vi "Update User Interface.vi"(8 "error in (no error)":errorcluster, 9 "VI Refnum":refnum<vi>, 11 "Data In":T1 {"Language" items=["English", "Español", "Português"]}) -> (0 "error out":errorcluster, 3 "Data Out":T1 {"Language" items=["English", "Español", "Português"]})   [LabVIEW 2017]
uses:
  Controls/HID Data.ctl
  <vilib>/userdefined/High Color/IMAQdx.ctl
  <vilib>/vision/Image Controls.llb/IMAQ Image.ctl
  Controls/HID State.ctl
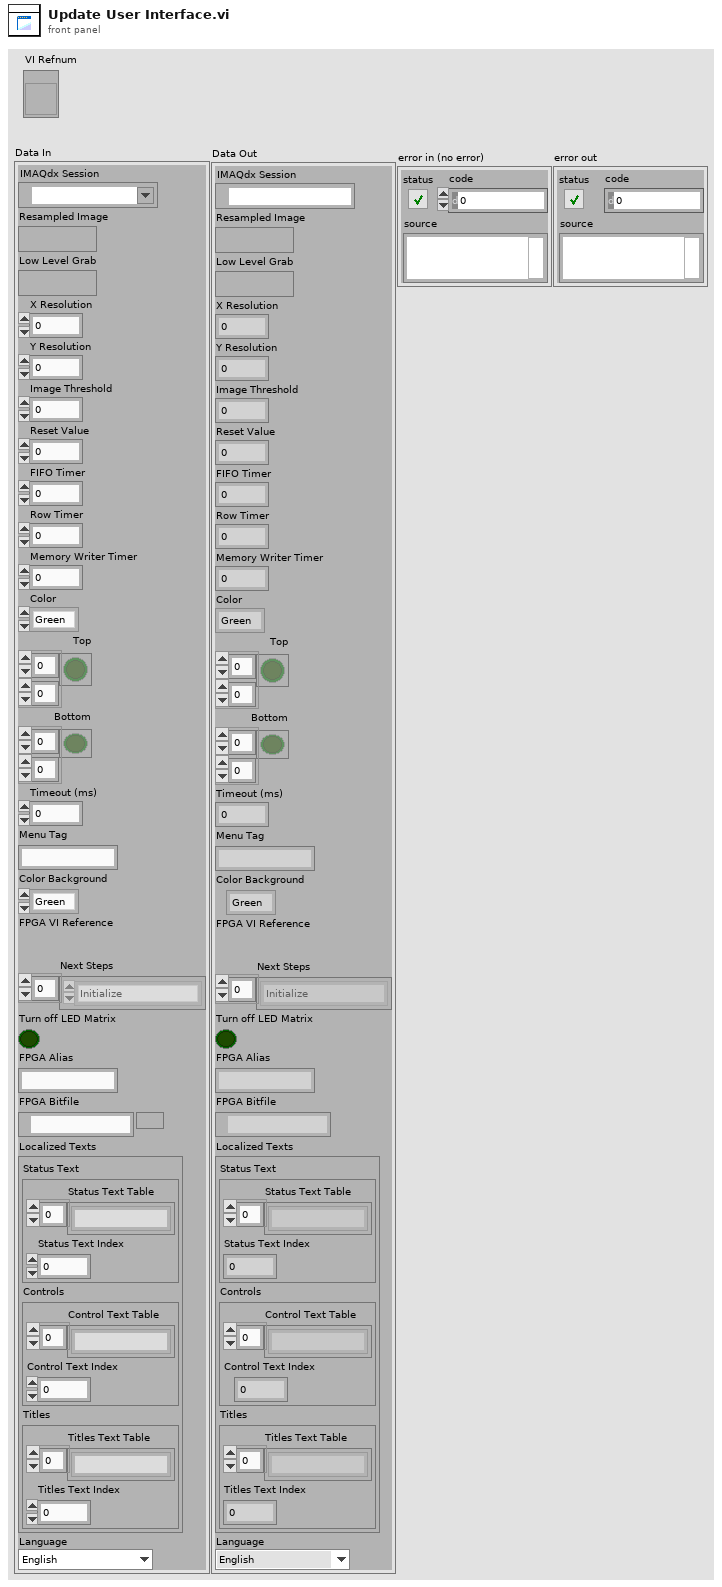
[diagram p1: front panel]
types:
  T1 = typedef "HID Data.ctl" = cluster{"IMAQdx Session":T2, "Resampled Image":T3, "Low Level Grab":T3, "X Resolution":i32, "Y Resolution":i32, "Image Threshold":u8, "Reset Value":i32, "FIFO Timer":u16, "Row Timer":u32, "Memory Writer Timer":u8, "Color":enum16{"Green", "Blue", "Red", "White", "Pink", "Yellow", "Turquoise", "Black"}, "Top":bool[][], "Bottom":bool[][], "Timeout (ms)":i32, "Menu Tag":string, "Color Background":enum16{"Green", "Blue", "Red", "White", "Pink", "Yellow", "Turquoise", "Black"}, "FPGA VI Reference":refnum<k20>, "Next Steps":T4[], "Turn off LED Matrix":bool, "FPGA Alias":string, "FPGA Bitfile":path, "Localized Texts":cluster{"Status Text":cluster{"Status Text Table":string[], "Status Text Index":i32}, "Controls":cluster{"Control Text Table":string[], "Control Text Index":i32}, "Titles":cluster{"Titles Text Table":string[], "Titles Text Index":i32}}, "Language":u16}
  T2 = typedef "IMAQdx.ctl" = refnum<k21>
  T3 = typedef "IMAQ Image.ctl" = refnum<image>
  T4 = typedef "HID State.ctl" = enum16{"Initialize", "Set FPGA Parametes", "Set Camera Parameters", "Set LED Matrix Parameters", "Initialize FPGA Interface", "Initialize Camera", "Start FPGA VI", "Start Camera", "Wait for Event", "Update UI", "Acquire", "Process Image", "Get Boolean Arrays", "Send to FPGA", "Menu Pop-Up", "Menu Actions", "Handle Errors", "Close Camera", "Close FPGA", "Stop", "Exit"}
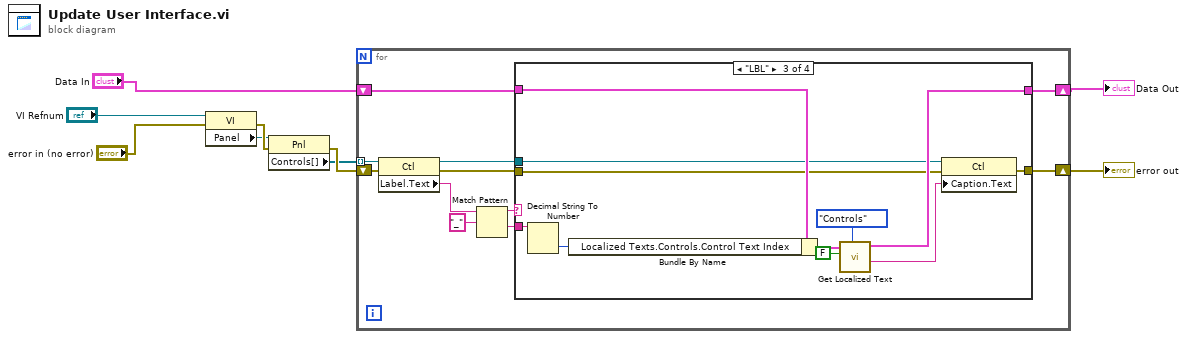
[diagram p0: block diagram]
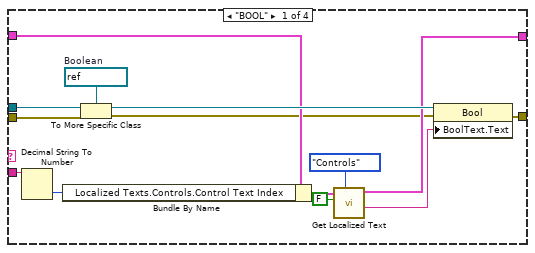
[diagram p2: hidden frame]
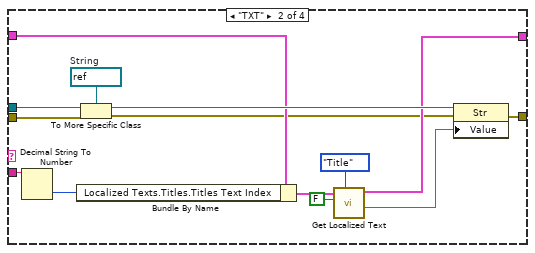
[diagram p3: hidden frame]
diagram:
  n1 = property class="VI"(reference="VI Refnum", error in="error in (no error)") -> (error out=w8:errorcluster, "Panel"=w6:refnum<vi>)  [unwired: 1 out]
  n2 = property class="Pnl"(reference=w6, error in=w8) -> (error out=w9:errorcluster, "Controls[]"=w5:refnum<vi>[])  [unwired: 1 out]
  n3 = for {
    tunnel: w5 -> [w18] mode=indexing
    shift-right: [w14] -> w3
    shift-left: "Data In" -> [w15]
    shift-right: [w11] -> w2
    shift-left: w9 -> [w10]
    n4 = property class="Ctl"(reference=w18, error in=w10) -> (reference out=w13:refnum<vi>, error out=w12:errorcluster, "Label.Text"=w17:string)
    n5 = Match Pattern(string=w17, regular expression="_") -> (before substring=w19:string, after substring=w16:string)  [unwired: 1 in, 2 out]
    n6 = case shown="\"LBL\"" w19 {
      tunnel: w16 -> [w32 w46 w59 _]
      tunnel: w15 -> [w29 w43 w56 w60]
      tunnel: [w28 w42 w55 w60] -> w14
      tunnel: w13 -> [w25 w39 w52 _]
      tunnel: w12 -> [w24 w38 w51 w61]
      tunnel: [w22 w36 w50 w61] -> w11
      frame "BOOL" {
        w33 = refnum<vi> refnum  # Boolean
        n7 = Decimal String To Number(string=w32) -> (number=w26:i32)  [unwired: 2 in, 1 out]
        n8 = Bundle By Name(cluster=w29, "Localized Texts.Controls.Control Text Index"=w26) -> (w27:T1)
        n9 = To More Specific Class(target class=w33, reference=w25, error in=w24) -> (specific class reference=w34:refnum<vi>, error out=w23:errorcluster)
        n10 = call "Get Localized Text.vi"("Text Type"=enum16{"Status", "Title", "Controls"}."Controls", "Force Index"=FALSE, "Data In"=w27) -> ("Localized Text"=w30:string, "Data Out"=w28:T1)  [unwired: 7 in]
        n11 = property class="Bool"(reference=w34, error in=w23, "BoolText.Text"=w30) -> (error out=w22:errorcluster)  [unwired: 1 out]
      }
      frame "TXT" {
        w47 = refnum<vi> refnum  # String
        n12 = Decimal String To Number(string=w46) -> (number=w40:i32)  [unwired: 2 in, 1 out]
        n13 = Bundle By Name(cluster=w43, "Localized Texts.Titles.Titles Text Index"=w40) -> (w41:T1)
        n14 = To More Specific Class(target class=w47, reference=w39, error in=w38) -> (specific class reference=w48:refnum<vi>, error out=w37:errorcluster)
        n15 = call "Get Localized Text.vi"("Text Type"=enum16{"Status", "Title", "Controls"}."Title", "Force Index"=FALSE, "Data In"=w41) -> ("Localized Text"=w44:string, "Data Out"=w42:T1)  [unwired: 7 in]
        n16 = property class="Str"(reference=w48, error in=w37, "Value"=w44) -> (error out=w36:errorcluster)  [unwired: 1 out]
      }
      frame "LBL" {
        n17 = Decimal String To Number(string=w59) -> (number=w53:i32)  [unwired: 2 in, 1 out]
        n18 = Bundle By Name(cluster=w56, "Localized Texts.Controls.Control Text Index"=w53) -> (w54:T1)
        n19 = call "Get Localized Text.vi"("Text Type"=enum16{"Status", "Title", "Controls"}."Controls", "Force Index"=FALSE, "Data In"=w54) -> ("Localized Text"=w57:string, "Data Out"=w55:T1)  [unwired: 7 in]
        n20 = property class="Ctl"(reference=w52, error in=w51, "Caption.Text"=w57) -> (error out=w50:errorcluster)  [unwired: 1 out]
      }
      frame "Any", Default {
      }
    }
  }
  "Data Out" <- w3
  "error out" <- w2
